vi "Add Step to Measurement Sequence.vi"(8 "error in (no error)":errorcluster, 10 "Step to Add":refnum<k7>, 11 "QPA Measurement in":refnum<class "QPA Measurement.lvclass">=refnum) -> (0 "error out":errorcluster, 3 "QPA Measurement out":refnum<class "QPA Measurement.lvclass">)   [LabVIEW 2016, in "QPA Measurement.lvlib" / "QPA Measurement.lvclass"]
uses:
  QPA Measurement.lvclass
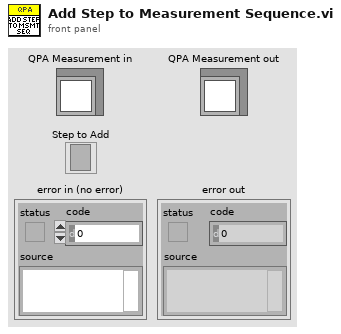
[diagram p1: front panel]
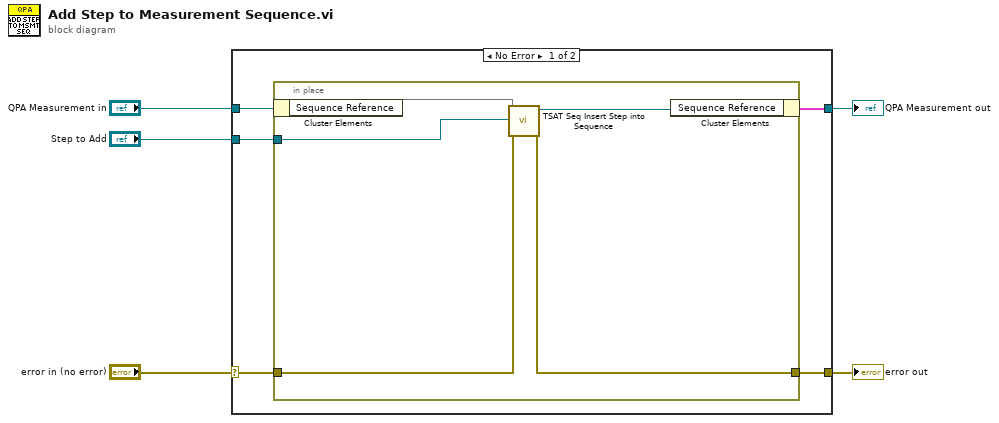
[diagram p0: block diagram]
diagram:
  n1 = case shown="No Error" "error in (no error)" {
    selector: "error in (no error)" -> [w8 w17]
    tunnel: [w7 w17] -> w4
    tunnel: [w9 w16] -> w2
    tunnel: "QPA Measurement in" -> [w10 w16]
    tunnel: "Step to Add" -> [w6 _]
    frame No Error {
      n2 = in-place {
        in-place-border: w8 -> [w13]
        in-place-border: [w12] -> w7
        in-place-border: w6 -> [w11]
        n3 = in-place-cluster #1(w10) -> ("Sequence Reference"=w15)
        n4 = call "TSAT Seq Insert Step into Sequence.vi"("Error in"=w13, "Step to Add"=w11, "Sequence In"=w15) -> ("error out"=w12:errorcluster, "Sequence Out"=w14:refnum<k7>)  [unwired: 7 in]
        n5 = in-place-cluster #1("Sequence Reference"=w14) -> (w9:cluster{})
      }
    }
    frame Error {
    }
  }
  "error out" <- w4
  "QPA Measurement out" <- w2
